vi "spark_max_pos_ctrl.vi"   [LabVIEW 2023]
uses:
  <vilib>/Rock Robotics/WPI/ThirdParty/REV Robotics/REVLib/SubVI/Public/SPARK Open Brushless.vi
  <vilib>/Rock Robotics/WPI/ThirdParty/REV Robotics/REVLib/SubVI/Public/SPARK Configure Basic Idle Mode.vi
  <vilib>/Rock Robotics/WPI/ThirdParty/REV Robotics/REVLib/SubVI/Public/SPARK Configure Power Smart Current Limit.vi
  <vilib>/Rock Robotics/WPI/ThirdParty/REV Robotics/REVLib/SubVI/Public/SPARK Configure Encoder Conversion Factors.vi
  <vilib>/Rock Robotics/WPI/ThirdParty/REV Robotics/REVLib/Typedef/Spark MAX Control Type.ctl
  <vilib>/Rock Robotics/WPI/ThirdParty/REV Robotics/REVLib/SubVI/Public/SPARK Get Alt Ext Encoder Status Position.vi
  <vilib>/Rock Robotics/WPI/ThirdParty/REV Robotics/REVLib/SubVI/Public/SPARK Get Device Status Applied Output.vi
  <vilib>/Rock Robotics/WPI/ThirdParty/REV Robotics/REVLib/SubVI/Public/SPARK Configure Closed Loop Basic.vi
  <vilib>/Rock Robotics/WPI/ThirdParty/REV Robotics/REVLib/SubVI/Public/SPARK Configure Absolute Encoder Basic.vi
  <vilib>/Rock Robotics/WPI/ThirdParty/REV Robotics/REVLib/SubVI/Public/SPARK Get Encoder Status Position.vi
  <vilib>/Rock Robotics/WPI/ThirdParty/REV Robotics/REVLib/SubVI/Public/SPARK Get Absolute Encoder Status Position.vi
types:
  T1 = typedef "Spark MAX Control Type.ctl" = enum16{"Percent VBus", "Voltage", "Velocity", "Position", "Smart Motion", "Current", "Smart Velocity", "MAXMotion Position", "MAXMotion Velocity"}
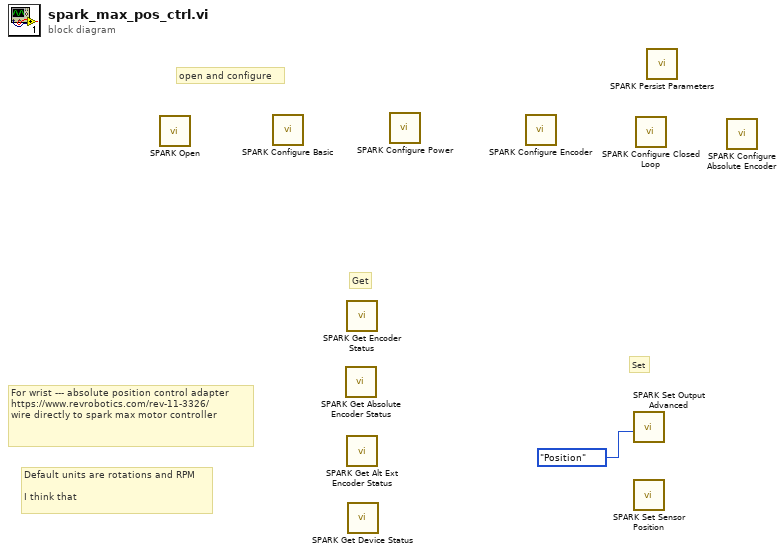
[diagram p0: block diagram]
diagram:
  # "Default units are rotations and RPM\n\nI think that"
  # "For wrist --- absolute position control adapter\nhttps://www.revrobotics.com/rev-11-3326/\nwire directly to spark max motor controller"
  # "open and configure"
  # "Set"
  # "Get"
  n1 = call-poly <vilib>:"SPARK Open.vi"() -> ()  [unwired: 10 in, 2 out]
  n2 = call-poly <vilib>:"SPARK Configure Basic.vi"() -> ()  [unwired: 10 in, 2 out]
  n3 = call-poly <vilib>:"SPARK Get Absolute Encoder Status.vi"() -> ()  [unwired: 8 in, 4 out]
  n4 = call-poly <vilib>:"SPARK Get Encoder Status.vi"() -> ()  [unwired: 8 in, 4 out]
  n5 = call-poly <vilib>:"SPARK Get Alt Ext Encoder Status.vi"() -> ()  [unwired: 8 in, 4 out]
  n6 = call-poly <vilib>:"SPARK Get Device Status.vi"() -> ()  [unwired: 8 in, 4 out]
  n7 = call-poly <vilib>:"SPARK Configure Power.vi"() -> ()  [unwired: 10 in, 2 out]
  n8 = call-poly <vilib>:"SPARK Configure Encoder.vi"() -> ()  [unwired: 10 in, 2 out]
  n9 = call <vilib>:"SPARK Set Output Advanced.vi"("Control Mode"=Spark_MAX_Control_Type."Position") -> ()  [unwired: 9 in, 2 out]
  n10 = call <vilib>:"SPARK Set Sensor Position.vi"() -> ()  [unwired: 10 in, 2 out]
  n11 = call-poly <vilib>:"SPARK Configure Closed Loop.vi"() -> ()  [unwired: 10 in, 2 out]
  n12 = call <vilib>:"SPARK Persist Parameters.vi"() -> ()  [unwired: 10 in, 2 out]
  n13 = call-poly <vilib>:"SPARK Configure Absolute Encoder.vi"() -> ()  [unwired: 10 in, 2 out]
